vi "Publish to Topic.vi"(8 "error in":errorcluster, 11 "Topic in":refnum<class "Topic.lvclass">) -> (0 "error out":errorcluster)   [LabVIEW 2014, in "Topic.lvclass"]
uses:
  Topic.lvclass
  Message_class/Message.lvclass
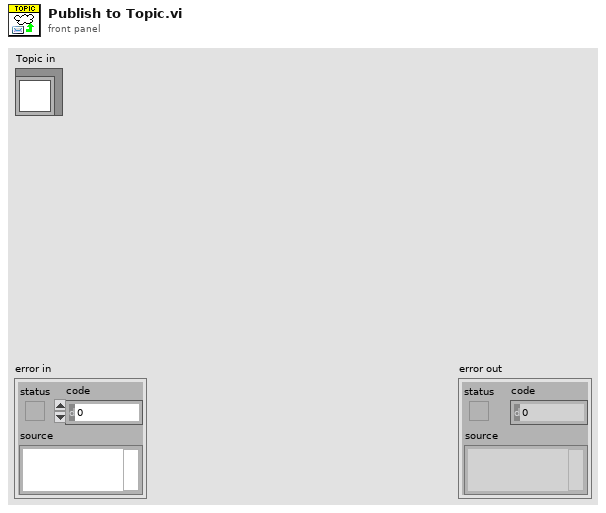
[diagram p1: front panel]
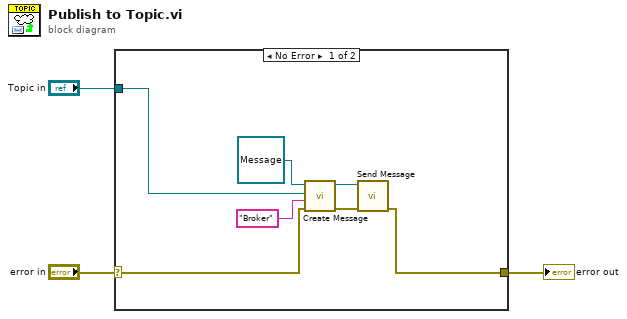
[diagram p0: block diagram]
diagram:
  n1 = case shown="No Error" "error in" {
    selector: "error in" -> [w5 w11]
    tunnel: [w4 w11] -> w2
    tunnel: "Topic in" -> [w6 _]
    frame No Error {
      n2 = call-dynamic "Create Message.vi"("error in"=w5, "Client ID"="Broker", "Topic.lvclass"=w6, "Message in"=refnum<class "Message.lvclass"> refnum ("Message.lvclass")) -> ("error out"=w10:errorcluster, "Message out"=w9:refnum<class "Message.lvclass">)  [unwired: 6 in]
      n3 = call-dynamic "Send Message.vi"("error in"=w10, "Message in"=w9) -> ("error out"=w4:errorcluster)  [unwired: 8 in, 1 out]
    }
    frame Error {
    }
  }
  "error out" <- w2
